vi "Hand_Store_Data_EMG_Control.vi"(10 "New Hand Positions":T3(array[cluster])) -> (2 "Hand motors info":T1(array[cluster]))   [LabVIEW 2015]
panel:
  in  "Cluster":T2
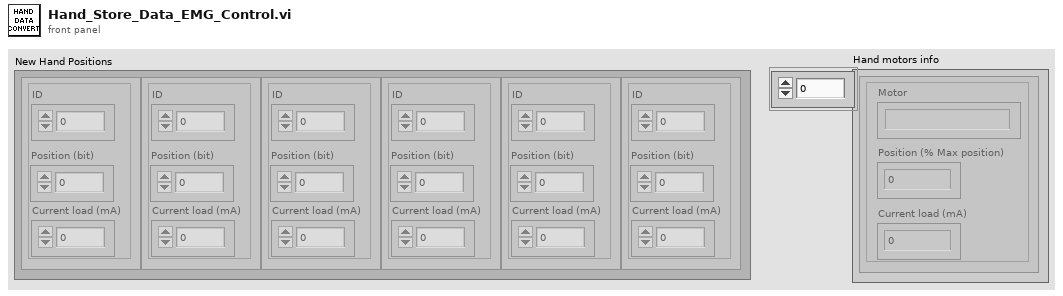
[diagram p1: front panel]
types:
  T1 = cluster{"Motor ":string, "Position (% Max position)":dbl, "Current load (mA)":dbl}[]
  T2 = cluster{"Motor ":string, "Position (% Max position)":dbl, "Current load (mA)":dbl}
  T3 = cluster{"ID":u16, "Position (bit)":u16, "Current load (mA)":u16}[]
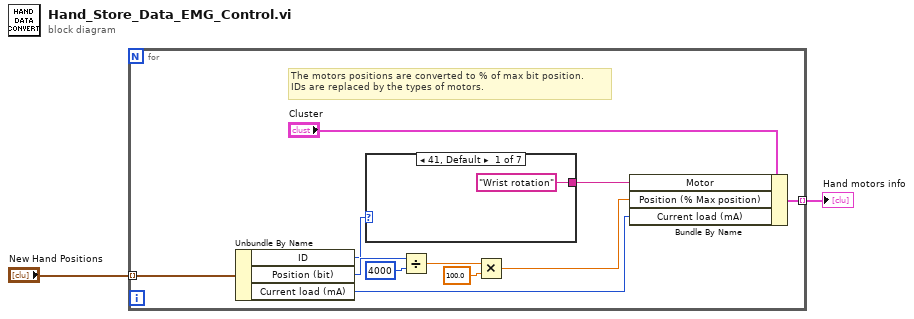
[diagram p0: block diagram]
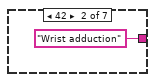
[diagram p2: hidden frame]
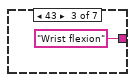
[diagram p3: hidden frame]
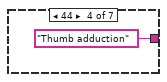
[diagram p4: hidden frame]
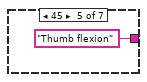
[diagram p5: hidden frame]
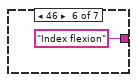
[diagram p6: hidden frame]
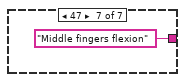
[diagram p7: hidden frame]
diagram:
  n1 = for {
    tunnel: "New Hand Positions" -> [w13] mode=indexing
    tunnel: [w3] -> w1 mode=indexing
    # "The motors positions are converted to % of max bit position.\nIDs are replaced by the types of motors."
    n2 = Unbundle By Name(w13) -> ("ID"=w8:u16, "Position (bit)"=w12:u16, "Current load (mA)"=w4:u16)
    n3 = case shown="41, Default" w8 {
      tunnel: ["Wrist rotation" "Wrist adduction" "Wrist flexion" "Thumb adduction" "Thumb flexion" "Index flexion" "Middle fingers flexion"] -> w5
      frame 41, Default {
      }
      frame 42 {
      }
      frame 43 {
      }
      frame 44 {
      }
      frame 45 {
      }
      frame 46 {
      }
      frame 47 {
      }
    }
    n4 = Divide(x=w12, y=u16 4000) -> (x/y=w11:dbl)
    n5 = Multiply(x=w11, y=100.0) -> (x*y=w6:dbl)
    n6 = Bundle By Name(cluster="Cluster", "Motor"=w5, "Position (% Max position)"=w6, "Current load (mA)"=w4) -> (w3:T2)
  }
  "Hand motors info" <- w1
